vi "Add Field.vi"(8 "error in (no error)":errorcluster, 10 "FieldSet":T1, 11 "DataPoint in":refnum<class "DataPoint.lvclass">) -> (0 "error out":errorcluster, 3 "DataPoint out":refnum<class "DataPoint.lvclass">)   [LabVIEW 2018, in "InfluxDB Client.lvlib" / "DataPoint.lvclass"]
uses:
  DataPoint.lvclass
  Controls/FieldSet.ctl
  DataPoint.lvclass/DataPoint.ctl
  InfluxDB Client.lvlib
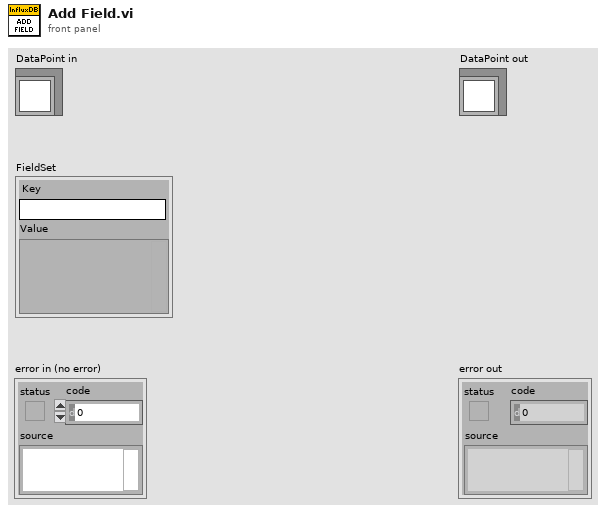
[diagram p1: front panel]
types:
  T1 = typedef "InfluxDB Client.lvlib/FieldSet.ctl" = cluster{"Key":string, "Value":variant}
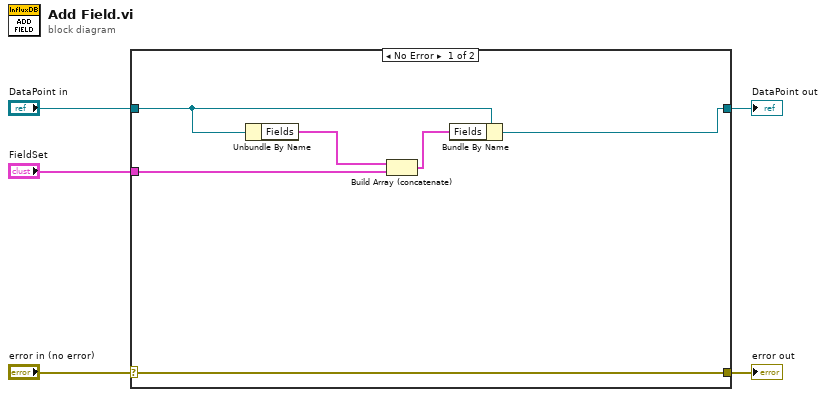
[diagram p0: block diagram]
diagram:
  n1 = case shown="No Error" "error in (no error)" {
    selector: "error in (no error)" -> [w11 w13]
    tunnel: [w11 w13] -> w4
    tunnel: "DataPoint in" -> [w8 w12]
    tunnel: "FieldSet" -> [w9 _]
    tunnel: [w6 w12] -> w1
    frame No Error {
      n2 = Unbundle By Name(w8) -> ("Fields"=w10:T1[])
      n3 = Build Array (concatenate)(w10, w9) -> (w7:T1[])
      n4 = Bundle By Name(cluster=w8, "Fields"=w7) -> (w6:refnum<class "DataPoint.lvclass">)
    }
    frame Error {
    }
  }
  "error out" <- w4
  "DataPoint out" <- w1
